vi "FTW-JSON-Duplicate.vi"(0 "JSON":T1, 11 "error in":errorcluster) -> (4 "JSON out":T1, 6 "Duplicated JSON":T1, 15 "error out":errorcluster)   [LabVIEW 2015]
uses:
  core/type/FTW-Type-JSON.ctl
panel:
  # "Inputs"
  # "Outputs"
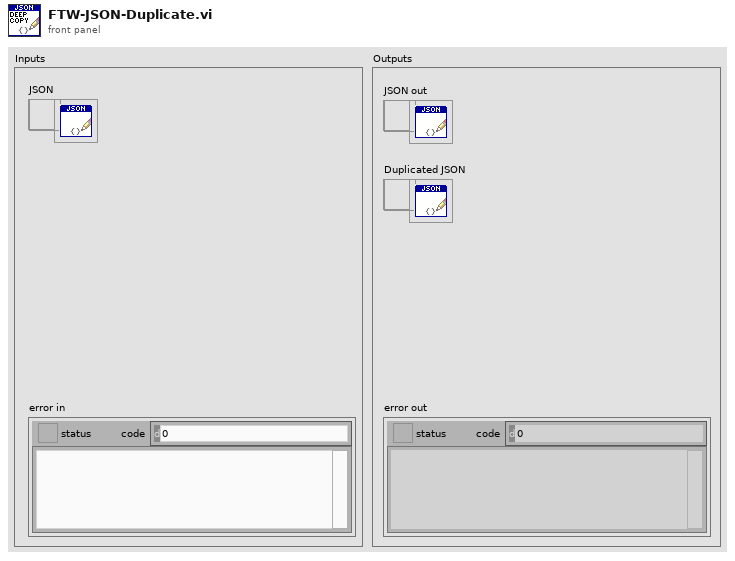
[diagram p1: front panel]
types:
  T1 = typedef "FTW-Type-JSON.ctl" = refnum<data-value>
  T2 = cluster{"FTW-CodeGen-Type":enum16{"FTW-JSON"}, "Object":i64, "EncodingFlags":i64, "DecodingFlags":i64}
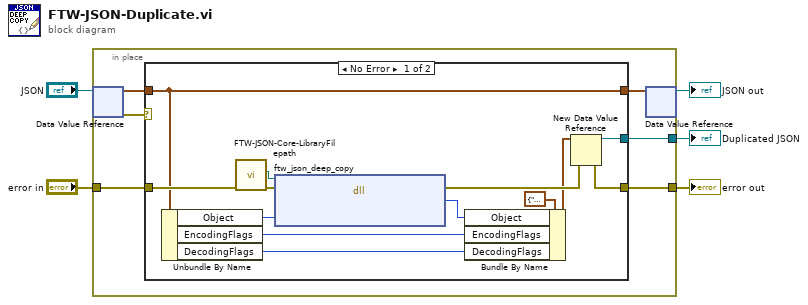
[diagram p0: block diagram]
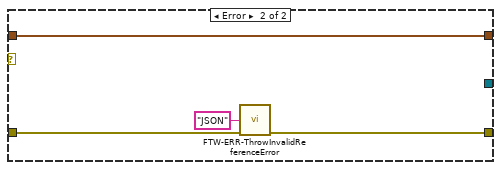
[diagram p2: hidden frame]
diagram:
  n1 = in-place {
    in-place-border: "error in" -> [w8]
    in-place-border: [w10] -> w5
    in-place-border: [w11] -> w1
    n2 = in-place-dvr #1("JSON") -> (w9:T2, w7:errorcluster)
    n3 = case shown="No Error" w7 {
      tunnel: [w20 _] -> w11
      tunnel: [w18 w26] -> w10
      tunnel: w9 -> [w12 w25]
      tunnel: w8 -> [w16 w27]
      tunnel: [w12 w25] -> w6
      frame No Error {
        n4 = Unbundle By Name(w12) -> ("Object"=w24:i64, "EncodingFlags"=w23:i64, "DecodingFlags"=w22:i64)
        n5 = call "FTW-JSON-Core-LibraryFilepath.vi"("error in"=w16) -> ("error out"=w15:errorcluster, "JSON Library Filepath"=w14:path)  [unwired: 9 in]
        n6 = dll-call lib="?" fn="ftw_json_deep_copy"(path in=w14, error in=w15, "Original JSON Object Pointer"=w24) -> (error out=w19:errorcluster, "Duplicate JSON Object Pointer"=w21:i64)  [unwired: 2 in, 1 out]
        n7 = Bundle By Name(cluster=T2 {"FTW-CodeGen-Type"=enum."FTW-JSON", "Object"=0, "EncodingFlags"=0, "DecodingFlags"=0}, "Object"=w21, "EncodingFlags"=w23, "DecodingFlags"=w22) -> (w17:T2)
        n8 = New Data Value Reference(data value=w17, error in=w19) -> (data value reference=w20:refnum<data-value>, error out=w18:errorcluster)
      }
      frame Error {
        n9 = call "FTW-ERR-ThrowInvalidReferenceError.vi"("Reference Type"="JSON", "error in"=w27) -> ("error out"=w26:errorcluster)  [unwired: 13 in]
      }
    }
    n10 = in-place-dvr #1(w6) -> (→"JSON out":T1)  [unwired: 1 out]
  }
  "error out" <- w5
  "Duplicated JSON" <- w1
